vi "SQL_Update.vi"(5 "To Update":string, 7 "Column Name":string, 8 "error in (no error)":errorcluster, 9 "Data":variant, 10 "Table":string, 11 "SQL in":refnum<class "SQL.lvclass">) -> (0 "error out":errorcluster, 3 "SQL out":refnum<class "SQL.lvclass">)   [LabVIEW 2012, in "SQL.lvclass"]
uses:
  SQL.lvclass
  <vilib>/addons/database/NI_Database_API.lvlib
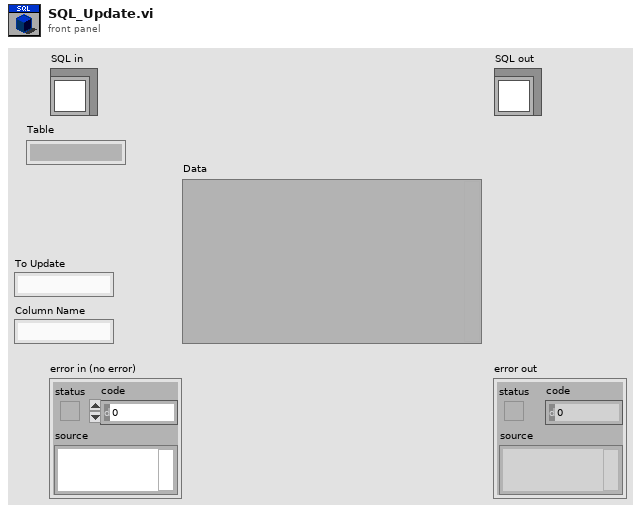
[diagram p1: front panel]
types:
  T1 = typedef "SQL.lvclass/ObjectAttributes.ctl" = cluster{"DB Connection Reference":T2}
  T2 = typedef "NI_Database_API.lvlib/Conn ObjectReference.ctl" = refnum<k1>
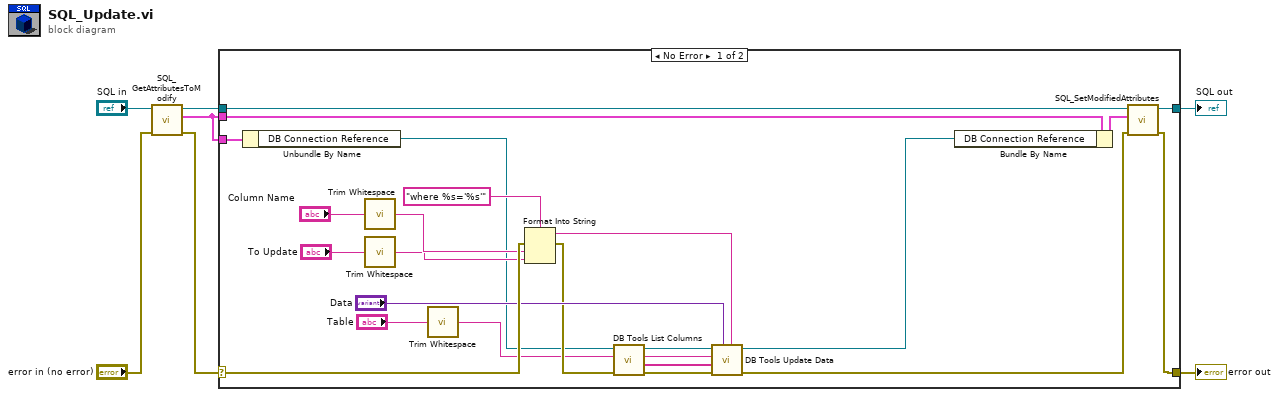
[diagram p0: block diagram]
diagram:
  n1 = call "SQL_GetAttributesToModify.vi"("error in (no error)"="error in (no error)", "reference in"="SQL in") -> ("error out"=w2:errorcluster, "Attributes"=w1:T1, "reference out"=w4:refnum<class "SQL.lvclass">)  [unwired: 6 in, 1 out]
  n2 = case shown="No Error" w2 {
    selector: w2 -> [w22 w32]
    tunnel: [w27 w32] -> w7
    tunnel: [w28 w31] -> w6
    tunnel: w4 -> [w29 w31]
    tunnel: w1 -> [w30 _]
    tunnel: w1 -> [w18 _]
    frame No Error {
      n3 = Unbundle By Name(w30) -> ("DB Connection Reference"=w11:T2)
      n4 = call <vilib>:"Trim Whitespace.vi"("string"="Column Name") -> ("trimmed string"=w15:string)  [unwired: 1 in]
      n5 = call <vilib>:"Trim Whitespace.vi"("string"="To Update") -> ("trimmed string"=w14:string)  [unwired: 1 in]
      n6 = call <vilib>:"Trim Whitespace.vi"("string"="Table") -> ("trimmed string"=w10:string)  [unwired: 1 in]
      n7 = Format Into String(format string="where %s='%s'", error in=w22, w15, w14) -> (resulting string=w23:string, error out=w13:errorcluster)  [unwired: 1 in]
      n8 = call <vilib>:"DB Tools List Columns.vi"("error in (no error)"=w13, "table"=w10, "connection reference"=w11) -> ("error out"=w12:errorcluster, "columns"=w8:string[], "connection reference out"=w9:T2)  [unwired: 1 in, 1 out]
      n9 = call <vilib>:"DB Tools Update Data.vi"("condition"=w23, "data"="Data", "error in (no error)"=w12, "columns"=w8, "table"=w10, "connection reference"=w9) -> ("error out"=w26:errorcluster, "connection reference out"=w16:T2)  [unwired: 4 in]
      n10 = Bundle By Name(cluster=w18, "DB Connection Reference"=w16) -> (w17:T1)
      n11 = call "SQL_SetModifiedAttributes.vi"("error in (no error)"=w26, "Attributes"=w17, "reference in"=w29) -> ("error out"=w27:errorcluster, "reference out"=w28:refnum<class "SQL.lvclass">)  [unwired: 7 in]
    }
    frame Error {
    }
  }
  "error out" <- w7
  "SQL out" <- w6
